vi "oa_FIR Preprocess Filter Order Checker.vi"(7 "filter types":T1(ring), 11 "order in":i32) -> (3 "order out":i32)   [LabVIEW 2017, in "SoundVib_RefDataProcess.lvlib"]
uses:
  <vilib>/addons/Sound and Vibration/Order Analysis/Referece Data Processing/SoundVib_RefDataProcess.lvlib
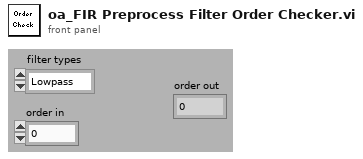
[diagram p1: front panel]
types:
  T1 = enum32{"Lowpass", "Highpass", "Bandpass", "Bandstop"}
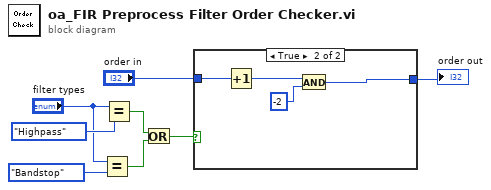
[diagram p0: block diagram]
diagram:
  n1 = Equal?(x="filter types", y=T1."Bandstop") -> (x = y?=w4:bool)
  n2 = Equal?(x="filter types", y=T1."Highpass") -> (x = y?=w5:bool)
  n3 = Or(x=w5, y=w4) -> (x .or. y?=w3:bool)
  n4 = case shown="True" w3 {
    tunnel: "order in" -> [w9 w13]
    tunnel: [w9 w11] -> w1
    frame False {
    }
    frame True {
      n5 = Increment(x=w13) -> (x+1=w10:i32)
      n6 = And(x=w10, y=-2) -> (x .and. y?=w11:i32)
    }
  }
  "order out" <- w1
